vi "RSZVB Read Receiver Power Correction Data.vi"(7 "Calibrated Wave":string, 8 "error in (no error)":errorcluster {"code" format="%.0x"}, 9 "Port Number (1)":i32=1, 10 "Channel (1)":i32=1, 11 "VISA session":refnum<visa-resource-name>) -> (0 "error out":errorcluster {"code" format="%.0x"}, 1 "Power Correction Values":dbl[](array[numeric]) format="%^.3e", 2 "Number Of Values":i32, 3 "dup VISA session":refnum<visa-resource-name>)   [LabVIEW 2011]
doc: "This VI reads receiver power correction data sets. \n\nNote(s):\n\n(1) A power correction data set contains n real values. Each value corresponds to the ratio of the actual power at the receiver input (value provided by the used source) to the uncalibrated power in dB. \n\n(2) The number n is equal to the number of sweep points.\n \n\nRemote-control command(s):\n[SENSe<Ch>:]CORRection:POWer<port_no>:DATA? '<wave_string>'"
uses:
  _utility/RSZVB Global Data.vi
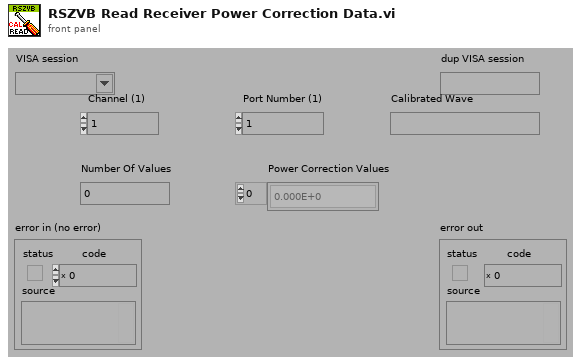
[diagram p1: front panel]
types:
  T1 = cluster{"Error Checking (T: On)":bool, "Installed Options":string[], "Data Valid?":bool, "Ports":i32, "Model":string[], "Option Checking (T: On)":bool}[]
  T2 = cluster{"Error Checking (T: On)":bool, "Installed Options":string[], "Data Valid?":bool, "Ports":i32, "Model":string[], "Option Checking (T: On)":bool}
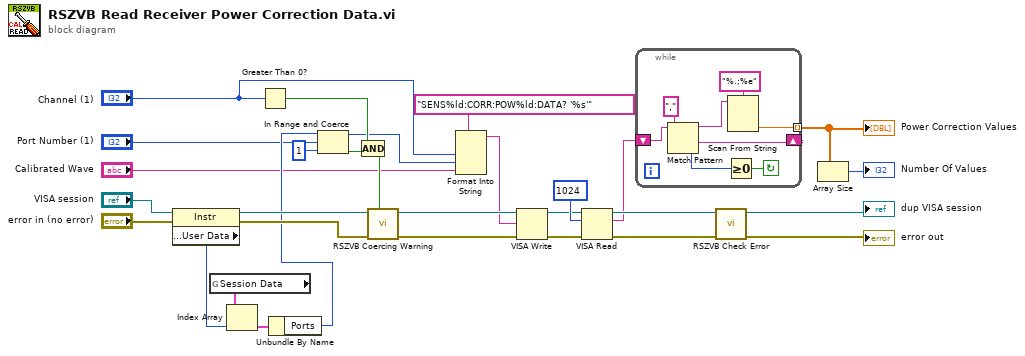
[diagram p0: block diagram]
diagram:
  n1 = property class="Instr"(reference="VISA session", error in="error in (no error)") -> (reference out=w22:refnum<visa-resource-name>, error out=w23:errorcluster, "General Settings:User Data"=w24:u32)
  n2 = global read "RSZVB Global Data.vi" "Session Data"() -> (w25:T1)
  n3 = Index Array(array=w25, index=w24) -> (element=w26:T2)
  n4 = Greater Than 0?(x="Channel (1)") -> (x > 0?=w28:bool)
  n5 = Unbundle By Name(w26) -> ("Ports"=w20:i32)
  n6 = In Range and Coerce(upper limit=w20, x="Port Number (1)", lower limit=1) -> (coerced(x)=w12:i32, In Range?=w19:bool)
  n7 = Compound Arithmetic op=AND(w28, w19) -> (w27:bool)
  n8 = call "RSZVB Coercing Warning.vi"("In Range?"=w27, "error in (no error)"=w23, "VISA session"=w22) -> ("error out"=w29:errorcluster, "dup VISA session"=w30:refnum<visa-resource-name>)  [unwired: 7 in]
  n9 = Format Into String(format string="SENS%ld:CORR:POW%ld:DATA? '%s'", "Channel (1)", w12, "Calibrated Wave") -> (resulting string=w11:string)  [unwired: 2 in, 1 out]
  n10 = VISA Write(VISA resource name=w30, write buffer=w11, error in (no error)=w29) -> (VISA resource name out=w14:refnum<visa-resource-name>, error out=w15:errorcluster)  [unwired: 1 out]
  n11 = VISA Read(VISA resource name=w14, byte count=u32 1024 ("byte count (0)"), error in (no error)=w15) -> (VISA resource name out=w18:refnum<visa-resource-name>, read buffer=w10:string, error out=w17:errorcluster)  [unwired: 1 out]
  n12 = while {
    shift-left: w10 -> [w36]
    shift-right: [w35] -> _
    tunnel: [w31] -> w6 mode=indexing
    stop <- w33 continue-if-true
    n13 = Match Pattern(string=w36, regular expression=",") -> (before substring=w34:string, after substring=w35:string, offset past match=w32:i32)  [unwired: 1 in, 1 out]
    n14 = Greater Or Equal To 0?(x=w32) -> (x >= 0?=w33:bool)
    n15 = Scan From String(format string="%.;%e", input string=w34) -> (output 1=w31:dbl)  [unwired: 3 in, 3 out]
  }
  "Power Correction Values" <- w6
  n16 = call "RSZVB Check Error.vi"("error in (no error)"=w17, "VISA session"=w18) -> ("error out"=→"error out":errorcluster, "dup VISA session"=→"dup VISA session":refnum<visa-resource-name>)  [unwired: 8 in]
  n17 = Array Size(array=w6) -> (size(s)=→"Number Of Values":i32)
